vi "Example.vi"(11 "CliArguments":string="-h") -> (0 "error out":errorcluster, 8 "StdErr":string, 9 "StdOut":string, 10 "Arguments":T1)   [LabVIEW 2022 SP3, in "ArgumentParser.lvlib"]
uses:
  ParsedData/_Arguments.ctl
  ParsedData/ParsedData.lvclass/ParsedData.ctl
  ParsedData/Read Arguments.vi
  ParsedData/Read StdErr.vi
  ParsedData/Read StdOut.vi
  ArgumentParser/ArgumentParser.lvclass
  ArgumentParser.lvlib
  ParsedData/ParsedData.lvclass
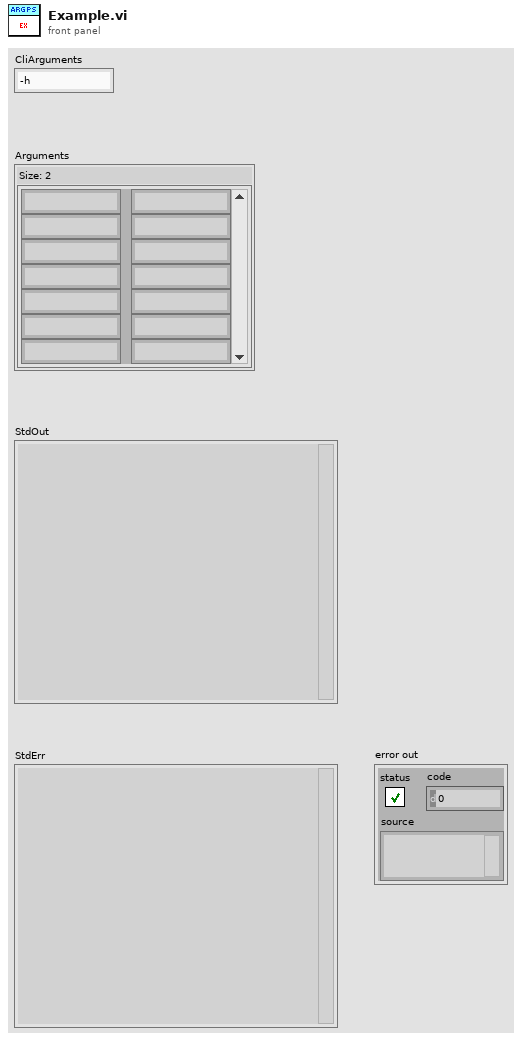
[diagram p1: front panel]
types:
  T1 = typedef "ArgumentParser.lvlib/ParsedData.lvclass/_Arguments.ctl" = map{string, string}
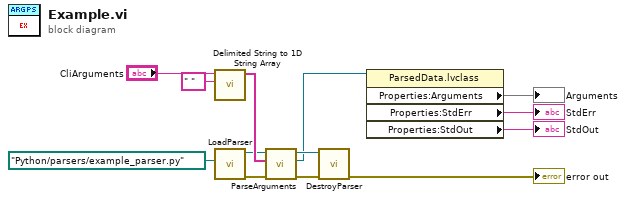
[diagram p0: block diagram]
diagram:
  n1 = call <vilib>:"Delimited String to 1D String Array.vi"("delimiter"=" ", "delimited string"="CliArguments") -> ("string array"=w7:string[])  [unwired: 9 in]
  n2 = call "LoadParser.vi"("ParserPath"=path "Python/parsers/example_parser.py" ("Path")) -> ("error out"=w12:errorcluster, "ArgumentParser"=w6:refnum<class "ArgumentParser.lvclass">)  [unwired: 9 in]
  n3 = call-dynamic "ParseArguments.vi"("error in (no error)"=w12, "CliArguments"=w7, "ArgumentParser in"=w6) -> ("error out"=w11:errorcluster, "ParsedData"=w4:refnum<class "ParsedData.lvclass">, "ArgumentParser out"=w10:refnum<class "ArgumentParser.lvclass">)  [unwired: 6 in]
  n4 = call-dynamic "DestroyParser.vi"("error in (no error)"=w11, "ArgumentParser in"=w10) -> ("error out"=→"error out":errorcluster)  [unwired: 9 in]
  n5 = property class="ParsedData.lvclass"(reference=w4) -> ("Properties:Arguments"=→"Arguments":T1, "Properties:StdErr"=→"StdErr":string, "Properties:StdOut"=→"StdOut":string)  [unwired: 1 in, 2 out]
